vi "Refresh with loaded ROI.vi"(7 "ROI fit info cluster":T1 {"ROI fit info"."Frame size"."Old" items=["100X100"=100, "128X128"=128, "200X200"=200, "256X256"=256, "512X512"=512, "1024x1024"=1024, "2048x2048"=2048]; "ROI fit info"."Frame size"."New" items=["100X100"=100, "128X128"=128, "200X200"=200, "256X256"=256, "512X512"=512, "1024x1024"=1024, "2048x2048"=2048]}, 10 "Old ROI file's data":dbl[][](array[numeric]), 11 "Old ROI file path":path) -> (1 "Last ROI Enum":T3, 3 "Proceed?":bool)   [LabVIEW 2020]
uses:
  Typedefs/ROI ID Enum.ctl
  Typedefs/ROI fitting info cluster.ctl
  Typedefs/Frame Size.ctl
  Typedefs/ROI management FG states.ctl
  Typedefs/Redraw ROI.ctl
panel:
  out "No ROI":bool
  out "Number of ROI":i32
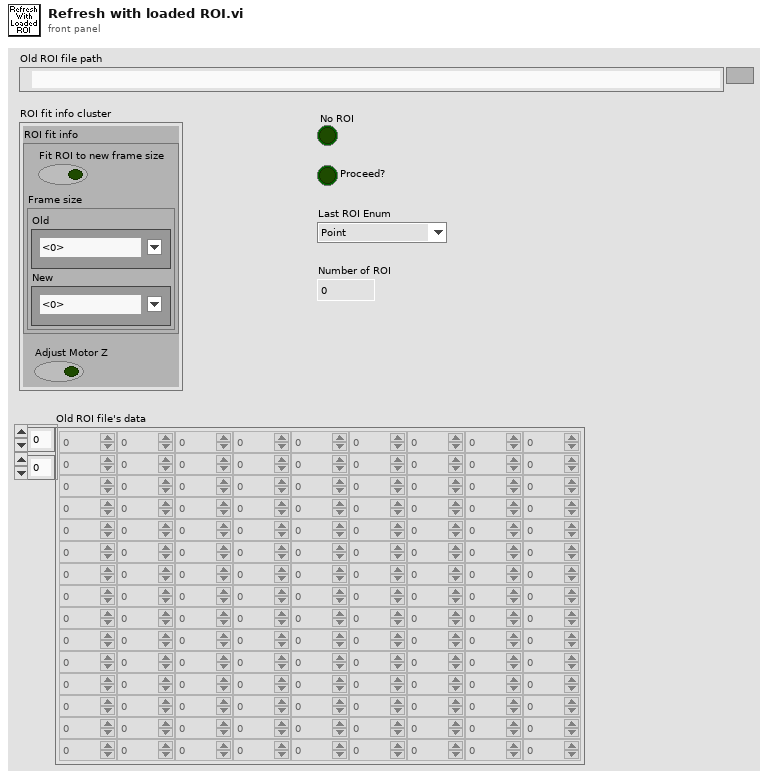
[diagram p1: front panel]
types:
  T1 = typedef "ROI fitting info cluster.ctl" = cluster{"ROI fit info":cluster{"Fit ROI to new frame size":bool, "Frame size":cluster{"Old":T2, "New":T2}}, "Adjust Motor Z":bool}
  T2 = typedef "Frame Size.ctl" = u16
  T3 = typedef "ROI ID Enum.ctl" = enum16{"Point", "MiniScan", "Comp. MiniScan", "Rectangle", "Comp. volume", "Arb. plane point", "None"}
  T4 = typedef "ROI management FG states.ctl" = enum16{"Read", "Write", "Write-from dataset", "Clear Last", "Clear All", "Delete ROI", "Update ROIs time", "Reload last ROI set", "Modify ROI Parameters", "Offset all ROI", "Offset visible ROI", "Modify Dwell Time", "Modify Laser Power"}
  T5 = typedef "Redraw ROI.ctl" = enum16{"Redraw All", "Redraw Deselected", "Draw Last", "Redraw Selected"}
  T6 = typedef "ROI spec.ctl" = cluster{"ROI Enum":T3, "Coordinates":i32[], "Zoom":dbl, "POI Dwell time":dbl, "Rel. Resolution":dbl, "Laser Power":dbl, "Frame Size":dbl, "FOV":dbl, "Z start":dbl, "Z stop":dbl, "Z planeIdx(s)":i32[], "Z planecodes(s)":u8[]}
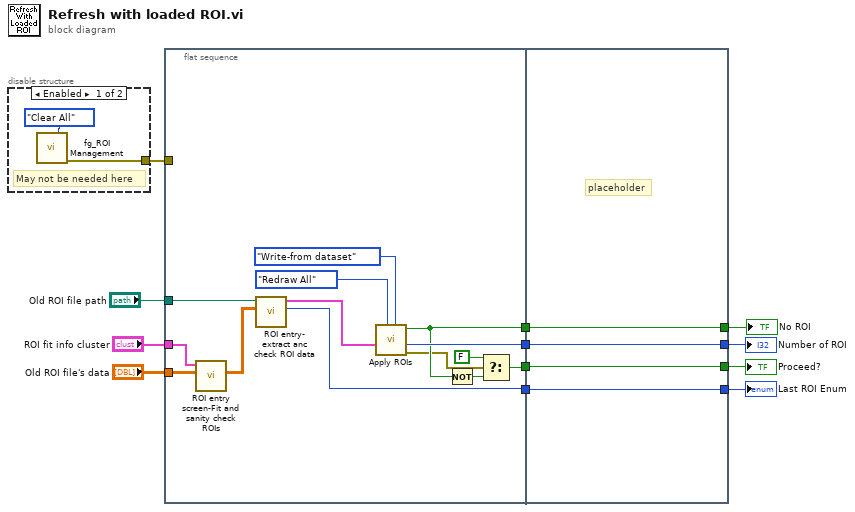
[diagram p0: block diagram]
diagram:
  n1 = disable-structure shown="Enabled" {
    disable-tunnel: [w13 _] -> w6
    frame Enabled {
      # "May not be needed here"
      n2 = call "fg_ROI Management.vi"("Function"=ROI_management_FG_states."Clear All") -> ("error out"=w13:errorcluster)  [unwired: 8 in, 6 out]
    }
    frame Disabled {
    }
  }
  n3 = flat-sequence {
    tunnel: "Old ROI file path" -> [w19]
    tunnel: "Old ROI file's data" -> [w25]
    tunnel: "ROI fit info cluster" -> [w24]
    tunnel: w6 -> [_]
    tunnel: [w28] -> w4
    tunnel: [w16] -> w3
    tunnel: [w27] -> w2
    tunnel: [w26] -> w1
    tunnel: [w29] -> w5
    tunnel: [w30] -> w9
    tunnel: [w31] -> w10
    tunnel: [w32] -> w11
    tunnel: w4 -> [w32]
    tunnel: w3 -> [w31]
    tunnel: w2 -> [w30]
    tunnel: w1 -> [w29]
    frame #0 {
      n4 = call "ROI entry screen-Fit and sanity check ROIs.vi"("Old ROI file's data in"=w25, "ROI fit info"=w24) -> ("Fitted ROI data"=w18:dbl[][])  [unwired: 9 in]
      n5 = call "ROI entry- extract anc check ROI data.vi"("ROI File data"=w18, "Old ROI file path"=w19) -> ("Last ROI Enum"=w16:T3, "Array"=w17:T6[])  [unwired: 5 in, 3 out]
      n6 = call "Apply ROIs.vi"("Function"=ROI_management_FG_states."Write-from dataset", "Mode (Redraw All)"=Redraw_ROI."Redraw All", "ROIs Info []"=w17) -> ("error out"=w22:errorcluster, "Number of ROI"=w27:i32, "No ROI"=w26:bool)  [unwired: 6 in]
      n7 = Not(x=w26) -> (.not. x?=w21:bool)
      n8 = Select(t=FALSE, s=w22, f=w21) -> (s? t:f=w28:bool)
    }
    frame #1 {
      # "placeholder"
    }
  }
  "Proceed?" <- w11
  "Last ROI Enum" <- w10
  "Number of ROI" <- w9
  "No ROI" <- w5
